vi "[GUIDELINE]SensorValuesToDashboard.vi"() -> ()   [LabVIEW 2019]
uses:
  <vilib>/Rock Robotics/Network Tables/NT Write Numeric Array.vi
  <vilib>/Rock Robotics/Network Tables/NT Write Boolean Array.vi
  <vilib>/Rock Robotics/Network Tables/NT Write String Array.vi
panel:
  in  "Slide":dbl(slide) scale=0.0..10.0
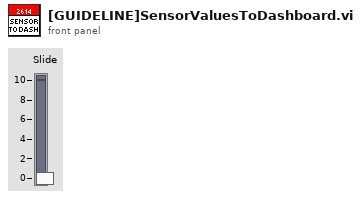
[diagram p1: front panel]
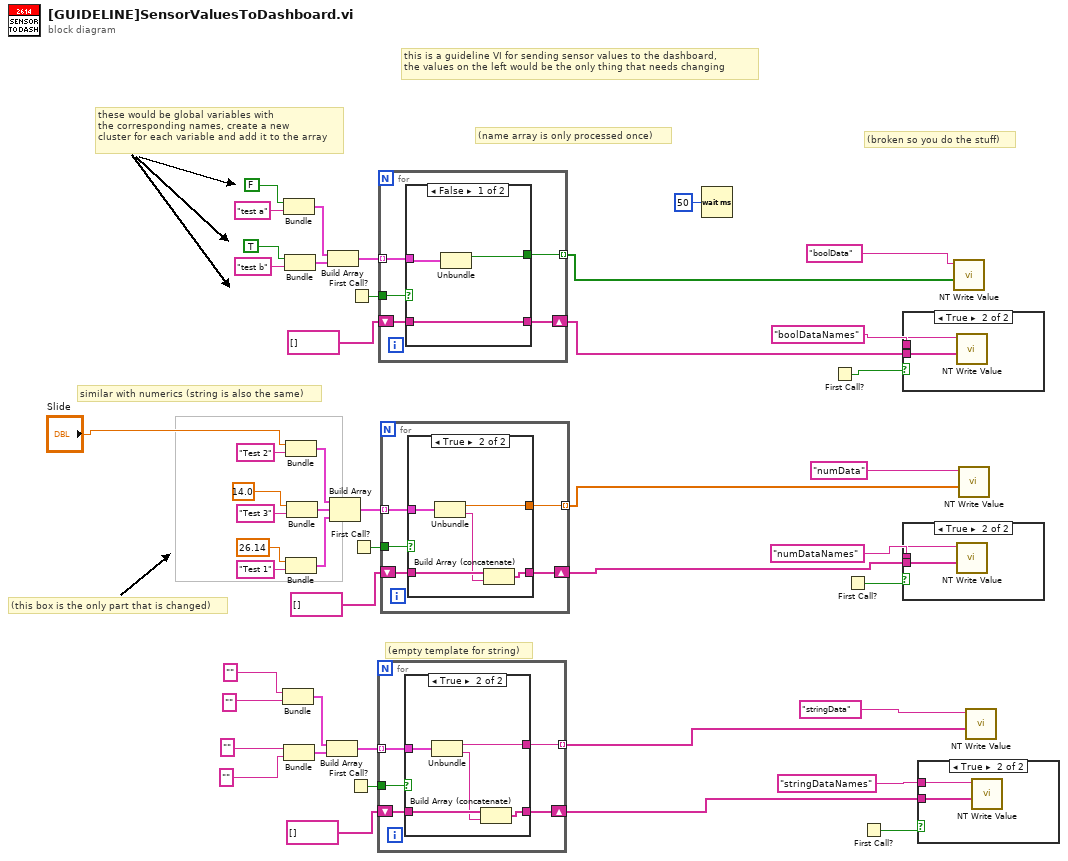
[diagram p0: block diagram]
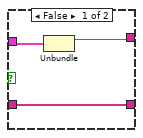
[diagram p5: hidden frame]
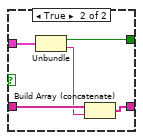
[diagram p6: hidden frame]
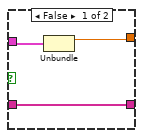
[diagram p7: hidden frame]
diagram:
  # "(empty template for string)"
  # "this is a guideline VI for sending sensor values to the dashboard, \nthe values on the left would be the only thing that needs changing"
  # "(broken so you do the stuff)"
  # "(this box is the only part that is changed)"
  # "(name array is only processed once)"
  # "similar with numerics (string is also the same)"
  # "these would be global variables with \nthe corresponding names, create a new\ncluster for each variable and add it to the array"
  n1 = Bundle("", "") -> (w13:cluster{string, string})  [unwired: 1 in]
  n2 = Bundle(FALSE, "test a") -> (w27:cluster{bool, string})  [unwired: 1 in]
  n3 = Bundle("", "") -> (w12:cluster{string, string})  [unwired: 1 in]
  n4 = Bundle(TRUE, "test b") -> (w21:cluster{bool, string})  [unwired: 1 in]
  n5 = Bundle("Slide"="Slide", "Test 2") -> (w22:cluster{"Slide":dbl, string})  [unwired: 1 in]
  n6 = Bundle("element"=26.14, "Test 1") -> (w40:cluster{"element":dbl, string})  [unwired: 1 in]
  n7 = Bundle("element"=14.0, "Test 3") -> (w41:cluster{"element":dbl, string})  [unwired: 1 in]
  n8 = Build Array(w13, w12) -> (w14:cluster{string, string}[])
  n9 = Build Array(w27, w21) -> (w28:cluster{bool, string}[])
  n10 = Build Array(w22, w41, w40) -> (w39:cluster{"element":dbl, string}[])
  n11 = First Call?() -> (First Call?: T/F=w16:bool)
  n12 = First Call?() -> (First Call?: T/F=w30:bool)
  n13 = First Call?() -> (First Call?: T/F=w37:bool)
  n14 = for {
    tunnel: w14 -> [w51] mode=indexing
    tunnel: [w50] -> w1 mode=indexing
    shift-right: [w48] -> w7
    shift-left: string[] [] -> [w49]
    tunnel: w16 -> [w47]
    n15 = case shown="True" w47 {
      tunnel: w51 -> [w54 w59]
      tunnel: [w53 w58] -> w50
      tunnel: w49 -> [w52 w57]
      tunnel: [w52 w55] -> w48
      frame False {
        n16 = Unbundle(w54) -> (w53:string)  [unwired: 1 out]
      }
      frame True {
        n17 = Unbundle(w59) -> (w58:string, w56:string)
        n18 = Build Array (concatenate)(w57, w56) -> (w55:string[])
      }
    }
  }
  n19 = for {
    tunnel: w28 -> [w64] mode=indexing
    tunnel: [w63] -> w20 mode=indexing
    shift-right: [w61] -> w19
    shift-left: string[] [] -> [w62]
    tunnel: w30 -> [w60]
    n20 = case shown="False" w60 {
      tunnel: w64 -> [w67 w72]
      tunnel: [w66 w71] -> w63
      tunnel: w62 -> [w65 w70]
      tunnel: [w65 w68] -> w61
      frame False {
        n21 = Unbundle(w67) -> (w66:bool)  [unwired: 1 out]
      }
      frame True {
        n22 = Unbundle(w72) -> (w71:bool, w69:string)
        n23 = Build Array (concatenate)(w70, w69) -> (w68:string[])
      }
    }
  }
  n24 = for {
    tunnel: w39 -> [w77] mode=indexing
    tunnel: [w76] -> w18 mode=indexing
    shift-right: [w74] -> w17
    shift-left: string[] [] -> [w75]
    tunnel: w37 -> [w73]
    n25 = case shown="True" w73 {
      tunnel: w77 -> [w80 w85]
      tunnel: [w79 w84] -> w76
      tunnel: w75 -> [w78 w83]
      tunnel: [w78 w81] -> w74
      frame False {
        n26 = Unbundle(w80) -> ("element"=w79:dbl)  [unwired: 1 out]
      }
      frame True {
        n27 = Unbundle(w85) -> ("element"=w84:dbl, w82:string)
        n28 = Build Array (concatenate)(w83, w82) -> (w81:string[])
      }
    }
  }
  n29 = Wait (ms)(milliseconds to wait=u32 50) -> ()  [unwired: 1 out]
  n30 = First Call?() -> (First Call?: T/F=w6:bool)
  n31 = First Call?() -> (First Call?: T/F=w5:bool)
  n32 = First Call?() -> (First Call?: T/F=w4:bool)
  n33 = case shown="True" w6 {
    tunnel: "boolDataNames" ("boolDataNames") -> [_ w87]
    tunnel: w19 -> [_ w86]
    frame False {
    }
    frame True {
      n34 = call-poly <vilib>:"NT Write Value.vi"("String Array"=w86, "Name"=w87) -> ()  [unwired: 9 in, 1 out]
    }
  }
  n35 = case shown="True" w5 {
    tunnel: "numDataNames" ("numDataNames") -> [_ w89]
    tunnel: w17 -> [_ w88]
    frame False {
    }
    frame True {
      n36 = call-poly <vilib>:"NT Write Value.vi"("String Array"=w88, "Name"=w89) -> ()  [unwired: 9 in, 1 out]
    }
  }
  n37 = case shown="True" w4 {
    tunnel: "stringDataNames" ("stringDataNames") -> [_ w91]
    tunnel: w7 -> [_ w90]
    frame False {
    }
    frame True {
      n38 = call-poly <vilib>:"NT Write Value.vi"("String Array"=w90, "Name"=w91) -> ()  [unwired: 9 in, 1 out]
    }
  }
  n39 = call-poly <vilib>:"NT Write Value.vi"("Boolean Array"=w20, "Name"="boolData" ("boolData")) -> ()  [unwired: 9 in, 1 out]
  n40 = call-poly <vilib>:"NT Write Value.vi"("Numeric Array"=w18, "Name"="numData" ("numData")) -> ()  [unwired: 9 in, 1 out]
  n41 = call-poly <vilib>:"NT Write Value.vi"("String Array"=w1, "Name"="stringData" ("stringData")) -> ()  [unwired: 9 in, 1 out]
